vi "Ballard XML Generator.Other Params.vi"(11 "other params":string[](array[string])) -> (3 "string":string)   [LabVIEW 2020]
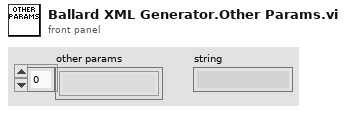
[diagram p1: front panel]
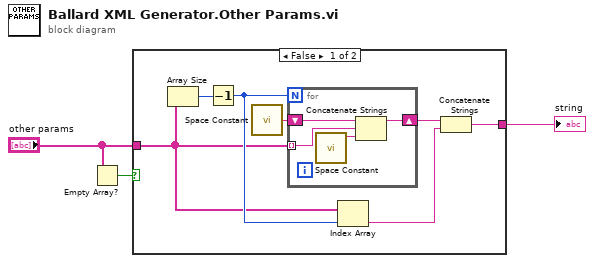
[diagram p0: block diagram]
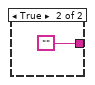
[diagram p2: hidden frame]
diagram:
  n1 = Empty Array?(array="other params") -> (empty?=w1:bool)
  n2 = case shown="False" w1 {
    tunnel: [w9 ""] -> w3
    tunnel: "other params" -> [w6 _]
    frame False {
      n3 = Array Size(array=w6) -> (size(s)=w5:i32)
      n4 = Decrement(x=w5) -> (x-1=w7:i32)
      n5 = call <vilib>:"Space Constant.vi"() -> ("String"=w4:string)
      n6 = for {
        N: w7 -> [_]
        tunnel: w6 -> [w13] mode=indexing
        shift-right: [w11] -> w8
        shift-left: w4 -> [w14]
        n7 = call <vilib>:"Space Constant.vi"() -> ("String"=w12:string)
        n8 = Concatenate Strings(w14, w13, w12) -> (w11:string)
      }
      n9 = Index Array(array=w6, index=w7) -> (element=w10:string)
      n10 = Concatenate Strings(w8, w10) -> (w9:string)
    }
    frame True {
    }
  }
  "string" <- w3
